vi "TimerEngine.GetWatchDog.vi"(8 "error in (no error)":errorcluster, 11 "DVR":refnum<data-value>) -> (0 "error out":errorcluster, 2 "WatchDog":T1, 3 "DVR 2":refnum<data-value>)   [LabVIEW 2017, in "TimerEngine.lvlib" / "TimerEngine.lvclass"]
uses:
  TimerEngine.lvclass
  _Typedef/WatchDog--QueueRef.ctl
  _Typedef/WatchDogData--Cluster.ctl
  _Typedef/Timer-UserEvent.ctl
  TimerEngine.lvclass/TimerEngine.ctl
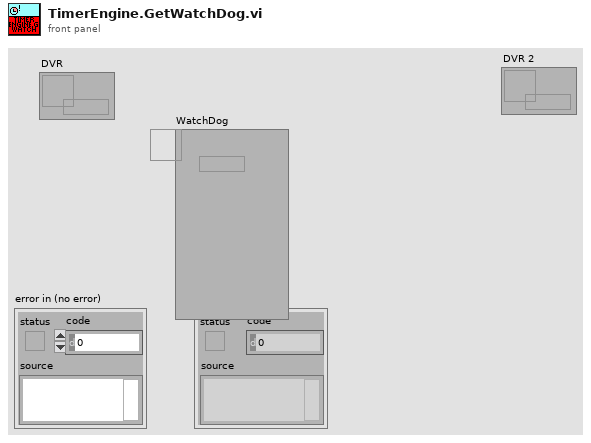
[diagram p1: front panel]
types:
  T1 = typedef "TimerEngine.lvlib/TimerEngine.lvclass/WatchDog--QueueRef.ctl" = refnum<queue>
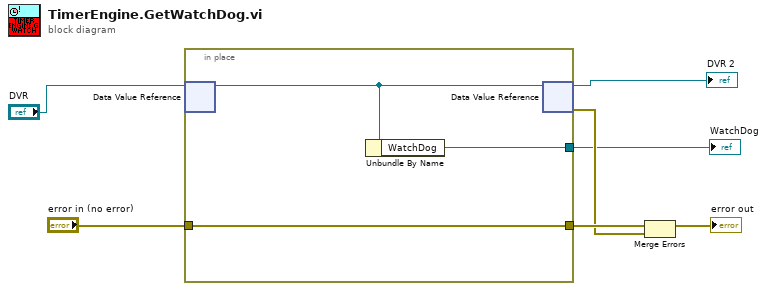
[diagram p0: block diagram]
diagram:
  n1 = in-place {
    in-place-border: [w10] -> w7
    in-place-border: "error in (no error)" -> [w10]
    in-place-border: [w8] -> w3
    n2 = in-place-dvr #1("DVR") -> (w9:refnum<class "TimerEngine.lvclass">)  [unwired: 1 out]
    n3 = Unbundle By Name(w9) -> ("WatchDog"=w8:T1)
    n4 = in-place-dvr #1(w9) -> (→"DVR 2":refnum<data-value>, w4:errorcluster)
  }
  "WatchDog" <- w3
  n5 = Merge Errors(w7, w4) -> (→"error out":errorcluster)
